vi "DataAcquisitionCode.vi"() -> ()   [LabVIEW 2020]
uses:
  globalvariables.vi
  <vilib>/Utility/file.llb/Read Delimited Spreadsheet (DBL).vi
panel:
  in  "ThM 4":enum32{"Page 1"}(tab)
  out "T-By In 4":dbl
  out "T-Hx In 4":dbl
  out "T-Supply 4":dbl
  out "P-Return 4":dbl
  out "T-Hx Out 4":dbl
  out "P-Hx Out 4":dbl
  out "T-By Out 4":dbl
  out "T-Return 4":dbl
  out "T-PJ Hot 4":dbl
  out "T-PJ Cold 4":dbl
  out "T-ThM 4":dbl(graph)
  out "P-Hx In 4":dbl
  out "P-By In 4":dbl
  out "M-Supply 4":dbl
  in  "ThM 3":enum32{"Page 1"}(tab)
  out "P-By In 3":dbl
  out "P-Hx In 3":dbl
  out "T-ThM 3":dbl(graph)
  out "T-PJ Cold 3":dbl
  out "T-PJ Hot 3":dbl
  out "T-Return 3":dbl
  out "T-By Out 3":dbl
  out "P-Return 3":dbl
  out "T-Hx Out 3":dbl
  out "P-Hx Out 3":dbl
  out "T-Supply 3":dbl
  out "T-By In 3":dbl
  out "T-Hx In 3":dbl
  out "M-Supply 3":dbl
  in  "ThM 1":enum32{"Page 1"}(tab)
  out "M-By 1":dbl format="%.2g"
  out "T-PJ Hot 1":dbl format="%.1g"
  out "T-PJ Cold 1":dbl format="%.1g"
  out "P-Hx Out 1":dbl format="%.2g"
  out "P-Hx In 1":dbl format="%.2g"
  out "P-By In 1":dbl format="%.2g"
  out "T-Hx Out 1":dbl format="%.1g"
  out "T-By Out 1":dbl format="%.1g"
  out "T-By In 1":dbl format="%.1g"
  out "T-Hx In 1":dbl format="%.1g"
  out "T-ThM 1":dbl(graph)
  in  "ThM 2":enum32{"Page 1"}(tab)
  out "M-By 2":dbl format="%.2g"
  out "T-Hx In 2":dbl format="%.1g"
  out "T-By In 2":dbl format="%.1g"
  out "T-Supply 2":dbl format="%.1g"
  out "P-Return 2":dbl format="%.2g"
  out "T-Return 2":dbl format="%.1g"
  out "P-Hx Out 2":dbl format="%.2g"
  out "T-By Out 2":dbl format="%.1g"
  out "T-Hx Out 2":dbl format="%.1g"
  out "T-PJ Hot 2":dbl format="%.1g"
  out "T-PJ Cold 2":dbl format="%.1g"
  out "T-ThM 2":dbl(graph)
  out "P-Hx In 2":dbl format="%.2g"
  out "P-By In 2":dbl format="%.2g"
  out "M-Supply 2":dbl format="%.2g"
  in  "Source":enum32{"Page 1"}(tab)
  out "T-Ambient":dbl format="%.1g"
  out "P-Pump In":dbl format="%.2g"
  out "T-Pump In":dbl format="%.1g"
  out "P-Heater Out":dbl format="%.2g"
  out "T-Heater Out":dbl format="%.1g"
  out "P-Heater In":dbl format="%.2g"
  out "M-Heater":dbl format="%.2g"
  out "T-Heater":dbl format="%.1g"
  in  "Heater Warning":enum32{"Page 1", "Page 2"}(tab)
  in  "Peltier Control Menu":enum32{"Cold Side", "Power"}(tab) caption="Peltier Control"
  in  "Run Peltier M":bool caption="Run"
  in  "Peltier Set Temp In":dbl[](array[slide]) step=0.1 scale=0.0..25.0
  in  "Peltier Update Rate":dbl=60.0 caption="Update Rate (s)"
  in  "Peltier Tamb In":dbl
  in  "Peltier Set Power":dbl[](array[numeric]) caption="Power Setpoint" format="%#.1f"
  out "Peltier Set Temp":dbl[](array[numeric]) caption="Control Temp" format="%#.1g"
  in  "Valve Control Menu":enum32{"Position", "PID"}(tab)
  in  "Run Valve M":bool caption="Run"
  in  "Valve Position Set":dbl[](array[knob]) min=0.0 max=100.0 step=0.1 scale=0.0..100.0
  in  "Valve Update Rate":dbl=60.0 caption="Update Rate (s)"
  in  "Valve Temp Setpoint":dbl[](array[numeric]) caption="Temp Setpoint"
  out "Valve Position":dbl[](array[numeric]) caption="Position"
  in  "Gain":cluster{"P":dbl, "I":dbl, "D":dbl}[](array[cluster]) caption="Gains"
  out "Time Elapsed (s)":dbl format="%#.0f"
  out "Time Limit (s)":dbl
  out "Current Save Directory":path
  out "# of Quick Restarts":i32
  out "# of Data Points Queued":i32
  out "Processing\nData":bool
  out "Acquiring\nData":bool
  in  "Stop Data Acquisition":bool
  # "Thermal Mass 4"
  # "Thermal Mass 3"
  # "Thermal Mass 1"
  # "Thermal Mass 2"
  # "Pump"
  # "Water Heater"
  # "WARNING:\nThe boiler has exceeded 90°C. Abort testing immediately."
  # "Peltier 1"
  # "Peltier 2"
  # "Valve 1"
  # "Valve 2"
  # "Valve 1"
  # "Valve 2"
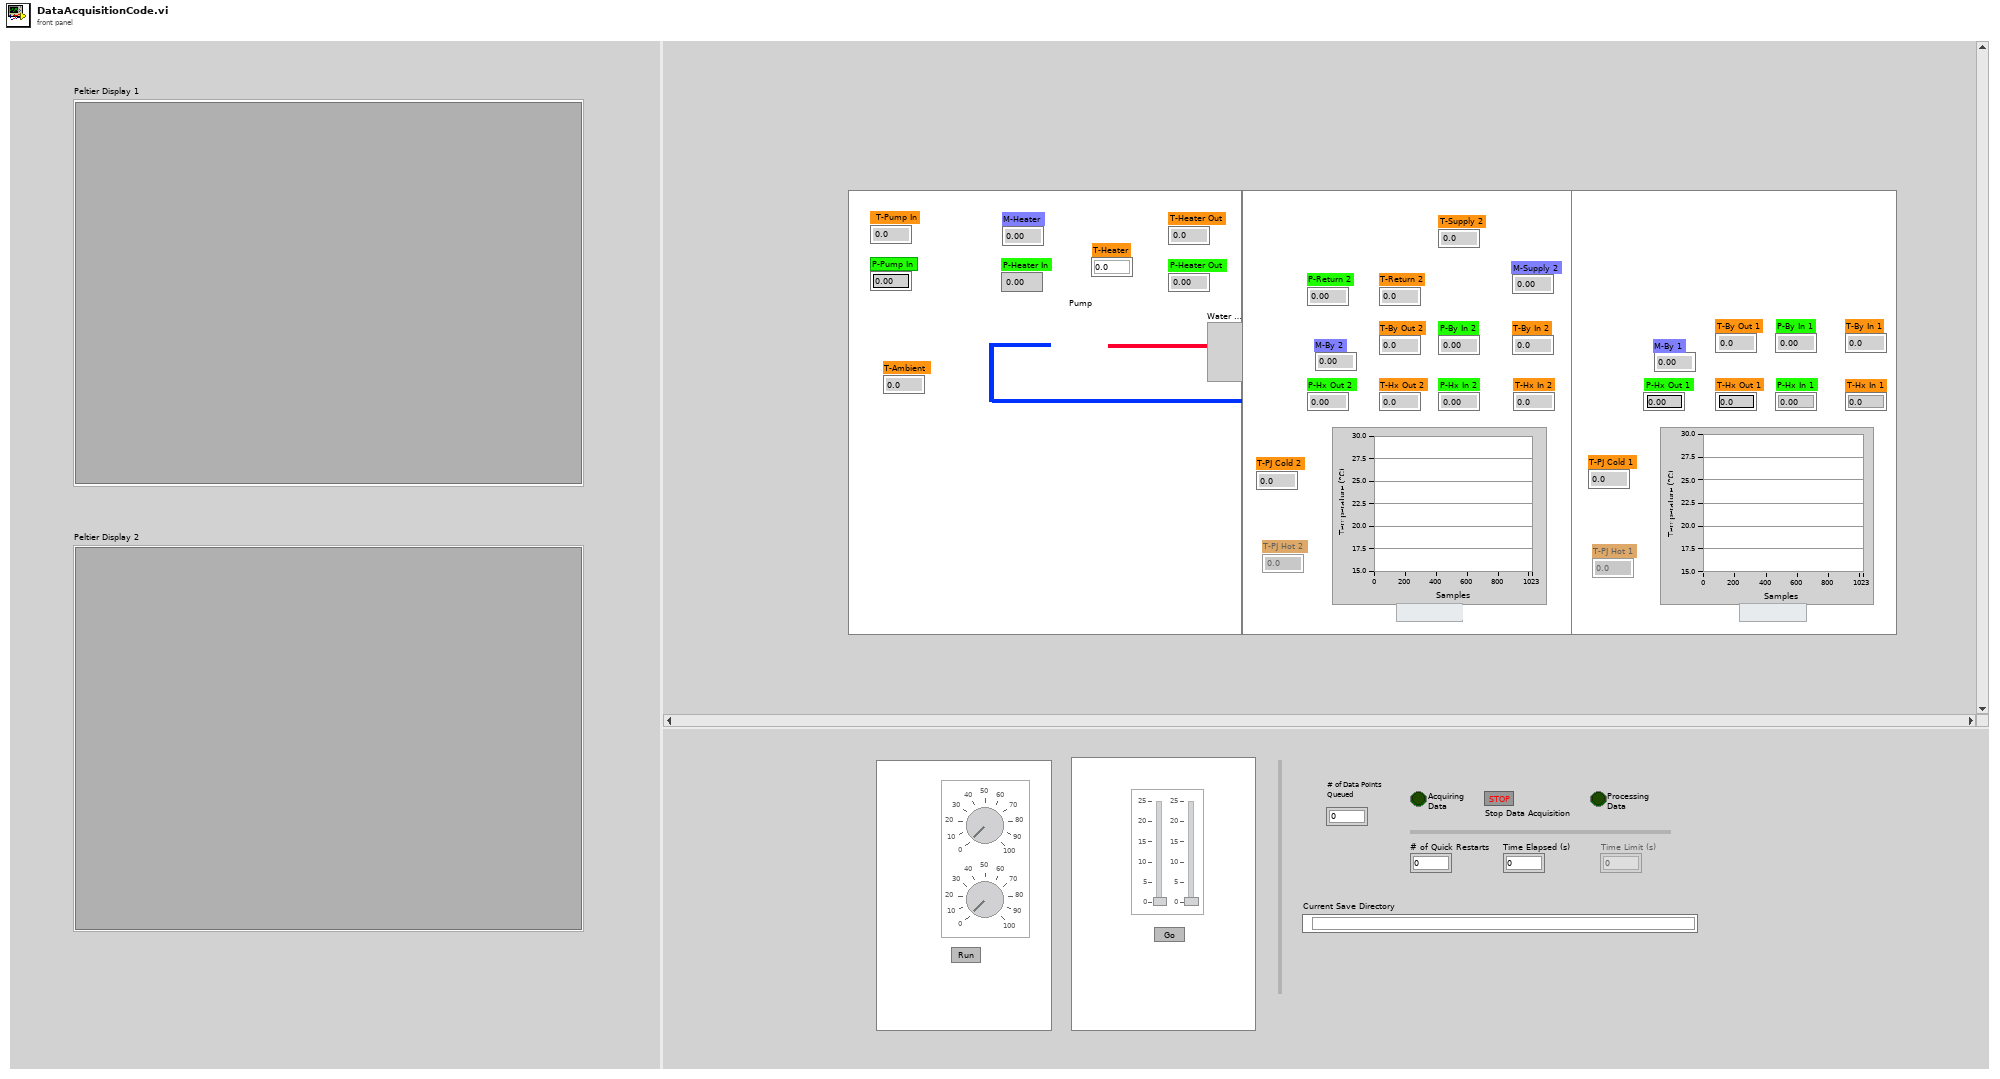
[diagram p1: front panel]
types:
  T1 = cluster{"Omega task":refnum<k24>[], "Sensor task":refnum<k21>, "Actuator task":refnum<k21>, "Omega error":errorcluster[], "Sensor error":errorcluster, "Actuator error":errorcluster}
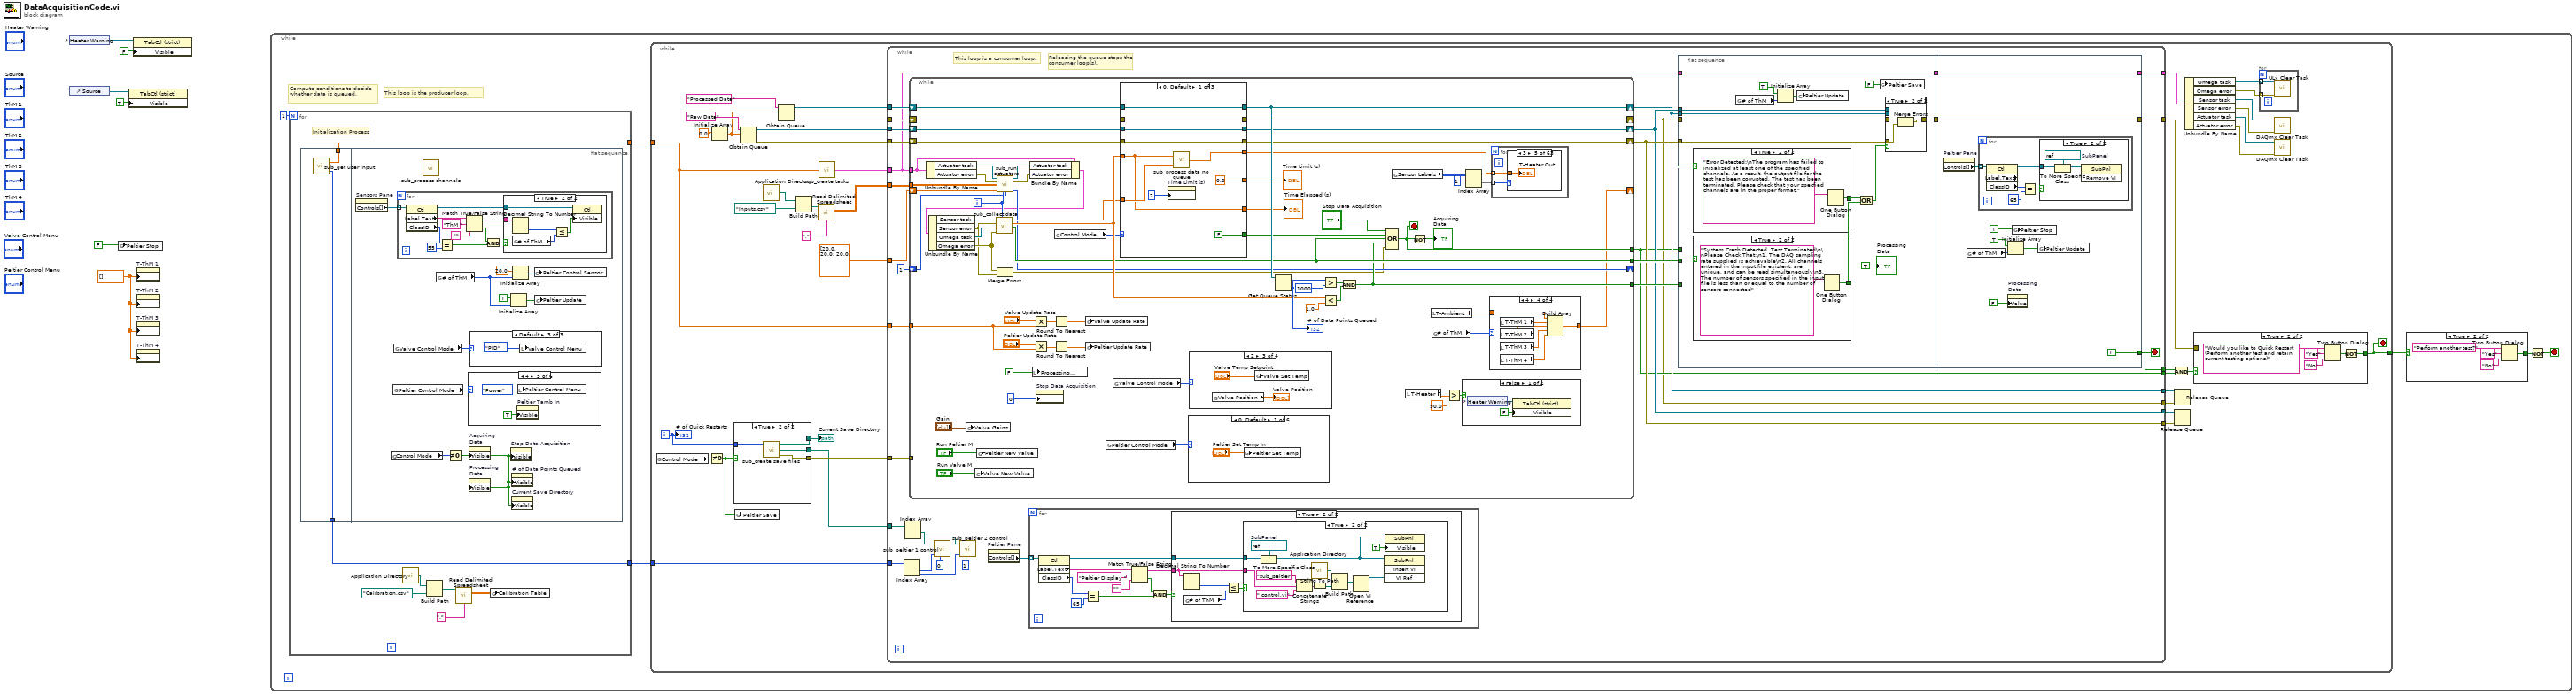
[diagram p0: block diagram]
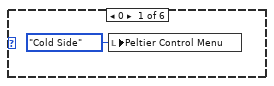
[diagram p3: hidden frame]
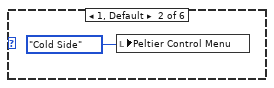
[diagram p4: hidden frame]
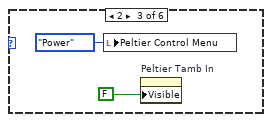
[diagram p5: hidden frame]
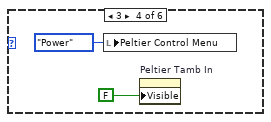
[diagram p6: hidden frame]
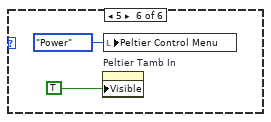
[diagram p7: hidden frame]
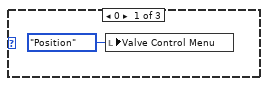
[diagram p8: hidden frame]
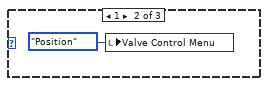
[diagram p9: hidden frame]
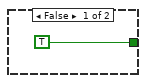
[diagram p10: hidden frame]
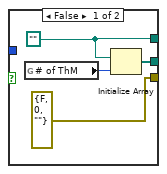
[diagram p11: hidden frame]
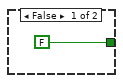
[diagram p12: hidden frame]
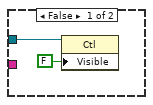
[diagram p14: hidden frame]
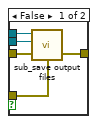
[diagram p15: hidden frame]
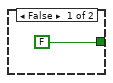
[diagram p16: hidden frame]
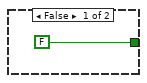
[diagram p17: hidden frame]
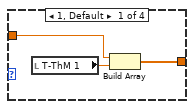
[diagram p19: hidden frame]
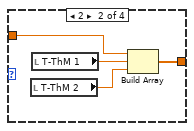
[diagram p20: hidden frame]
diagram:
  w2 = dbl[] []
  n1 = control-ref of="Heater Warning"() -> (w5:refnum<vi>)
  n2 = control-ref of="Source"() -> (w4:refnum<vi>)
  n3 = global write "globalvariables.vi" "Peltier Stop"(FALSE) -> ()
  n4 = property on="Property Node" class="TabCtl (strict)"(reference=w4, "Visible"=TRUE) -> ()  [unwired: 1 in, 2 out]
  n5 = property on="Property Node" class="TabCtl (strict)"(reference=w5, "Visible"=FALSE) -> ()  [unwired: 1 in, 2 out]
  n6 = property on="T-ThM 1" class="WFChart (strict)"("History Data"=w2) -> ()  [unwired: 2 in, 2 out]
  n7 = property on="T-ThM 2" class="WFChart (strict)"("History Data"=w2) -> ()  [unwired: 2 in, 2 out]
  n8 = property on="T-ThM 3" class="WFChart (strict)"("History Data"=w2) -> ()  [unwired: 2 in, 2 out]
  n9 = property on="T-ThM 4" class="WFChart (strict)"("History Data"=w2) -> ()  [unwired: 2 in, 2 out]
  n10 = while {
    stop <- w11 stop-if-true
    # "Compute conditions to decide whether data is queued."
    # "This loop is the producer loop."
    n11 = for {
      N: 1 -> [_]
      tunnel: [w19] -> w9
      tunnel: [w13] -> w7
      # "Initialization Process"
      n12 = flat-sequence {
        tunnel: [w21] -> w19
        tunnel: [w20] -> w13
        frame #0 {
          n13 = call "sub_get user input.vi"() -> ("Peltier Channels"=w20:i16[], "DAQ Sample Rate"=w21:dbl)  [unwired: 2 in]
        }
        frame #1 {
          n14 = property on="Sensors Pane" class="Pane"() -> ("Controls[]"=w22:refnum<vi>[])  [unwired: 2 in, 2 out]
          n15 = global read "globalvariables.vi" "Control Mode"() -> (w28:i32)
          n16 = global read "globalvariables.vi" "Peltier Control Mode"() -> (w30:i16)
          n17 = global read "globalvariables.vi" "Valve Control Mode"() -> (w31:i16)
          n18 = for {
            tunnel: w22 -> [w40] mode=indexing
            n19 = property class="Ctl"(reference=w40) -> (reference out=w41:refnum<vi>, "Label.Text"=w39:string, "ClassID"=w42:u32)  [unwired: 1 in, 1 out]
            n20 = Equal?(x=w42, y=u32 55) -> (x = y?=w32:bool)
            n21 = Match True/False String(2:"", 3:"ThM " ("true string"), 4:w39) -> (0:w33:bool, 1:w35:string)
            n22 = And(x=w33, y=w32) -> (x .and. y?=w34:bool)
            n23 = case shown="True" w34 {
              tunnel: w41 -> [_ w47]
              tunnel: w35 -> [_ w46]
              frame False {
              }
              frame True {
                n24 = global read "globalvariables.vi" "# of ThM"() -> (w43:i32)
                n25 = Decimal String To Number(string=w46) -> (number=w44:i32)  [unwired: 2 in, 1 out]
                n26 = Less Or Equal?(x=w44, y=w43) -> (x <= y?=w45:bool)
                n27 = property class="Ctl"(reference=w47, "Visible"=w45) -> ()  [unwired: 1 in, 2 out]
              }
            }
          }
          n28 = call "sub_process channels.vi"() -> ()  [unwired: 6 in]
          n29 = global read "globalvariables.vi" "# of ThM"() -> (w24:i32)
          n30 = Not Equal To 0?(x=w28) -> (x != 0?=w29:bool)
          n31 = case shown="4" w30 {
            frame 0 {
              n32 = local write "Peltier Control Menu"(enum32{"Cold Side", "Power"}."Cold Side" ("Peltier Control Menu")) -> ()
            }
            frame 1, Default {
              n33 = local write "Peltier Control Menu"(enum32{"Cold Side", "Power"}."Cold Side" ("Peltier Control Menu")) -> ()
            }
            frame 2 {
              n34 = local write "Peltier Control Menu"(enum32{"Cold Side", "Power"}."Power" ("Peltier Control Menu")) -> ()
              n35 = property on="Peltier Tamb In" class="DigNum (strict)"("Visible"=FALSE) -> ()  [unwired: 2 in, 2 out]
            }
            frame 3 {
              n36 = local write "Peltier Control Menu"(enum32{"Cold Side", "Power"}."Power" ("Peltier Control Menu")) -> ()
              n37 = property on="Peltier Tamb In" class="DigNum (strict)"("Visible"=FALSE) -> ()  [unwired: 2 in, 2 out]
            }
            frame 4 {
              n38 = property on="Peltier Tamb In" class="DigNum (strict)"("Visible"=TRUE) -> ()  [unwired: 2 in, 2 out]
              n39 = local write "Peltier Control Menu"(enum32{"Cold Side", "Power"}."Power" ("Peltier Control Menu")) -> ()
            }
            frame 5 {
              n40 = property on="Peltier Tamb In" class="DigNum (strict)"("Visible"=TRUE) -> ()  [unwired: 2 in, 2 out]
              n41 = local write "Peltier Control Menu"(enum32{"Cold Side", "Power"}."Power" ("Peltier Control Menu")) -> ()
            }
          }
          n42 = property on="Acquiring\nData" class="Bool (strict)"("Visible"=w29) -> ()  [unwired: 2 in, 2 out]
          n43 = property on="Processing\nData" class="Bool (strict)"("Visible"=w29) -> ()  [unwired: 2 in, 2 out]
          n44 = case shown="Default" w31 {
            frame 0 {
              n45 = local write "Valve Control Menu"(enum32{"Position", "PID"}."Position" ("Valve Control Menu")) -> ()
            }
            frame 1 {
              n46 = local write "Valve Control Menu"(enum32{"Position", "PID"}."Position" ("Valve Control Menu")) -> ()
            }
            frame Default {
              n47 = local write "Valve Control Menu"(enum32{"Position", "PID"}."PID" ("Valve Control Menu")) -> ()
            }
          }
          n48 = Initialize Array(TRUE, w24) -> (w23:bool[])
          n49 = property on="Stop Data Acquisition" class="Bool"("Visible"=w29) -> ()  [unwired: 2 in, 2 out]
          n50 = property on="# of Data Points Queued" class="DigNum (strict)"("Visible"=w29) -> ()  [unwired: 2 in, 2 out]
          n51 = property on="Current Save Directory" class="Path"("Visible"=w29) -> ()  [unwired: 2 in, 2 out]
          n52 = Initialize Array(20.0 ("element"), w24) -> (w26:dbl[])
          n53 = global write "globalvariables.vi" "Peltier Control Sensor"(w26) -> ()
          n54 = global write "globalvariables.vi" "Peltier Update"(w23) -> ()
        }
      }
      n55 = call <vilib>:"Application Directory.vi"() -> ("Application Directory"=w17:path)
      n56 = Build Path(base path=w17, name or relative path=path "Calibration.csv") -> (appended path=w18:path)
      n57 = call-poly <vilib>:"Read Delimited Spreadsheet.vi"("file path (dialog if empty)"=w18, "delimiter (\\t)"=",") -> ("all rows"=w16:dbl[][])  [unwired: 8 in, 5 out]
      n58 = global write "globalvariables.vi" "Calibration Table"(w16) -> ()
    }
    n59 = while {
      tunnel: [w99] -> w10
      tunnel: w9 -> [w92]
      tunnel: w7 -> [w67]
      i -> [w90]
      stop <- w99 stop-if-true
      n60 = global read "globalvariables.vi" "Control Mode"() -> (w88:i32)
      n61 = Not Equal To 0?(x=w88) -> (x != 0?=w87:bool)
      n62 = Initialize Array(0.0) -> (w84:dbl[])  [unwired: 1 in]
      n63 = case shown="True" w87 {
        tunnel: w90 -> [_ w112]
        tunnel: [w108 w111] -> w73
        tunnel: [errorcluster {"status"=FALSE, "code"=0, "source"=""} ("error constant") w110] -> w86
        tunnel: [w105 w109] -> w81
        frame False {
          w105 = path ""
          n64 = global read "globalvariables.vi" "# of ThM"() -> (w107:i32)
          n65 = Initialize Array(w105, w107) -> (w108:path[])
        }
        frame True {
          n66 = call "sub_create save files.vi"("# of Quick Restarts"=w112) -> ("error out"=w110:errorcluster, "Peltier Save Files"=w111:path[], "Save Path"=w109:path)  [unwired: 2 in]
        }
      }
      "Current Save Directory" <- w81
      n67 = global write "globalvariables.vi" "Peltier Save"(w87) -> ()
      n68 = Obtain Queue(name (unnamed)="Raw Data", element data type=w84) -> (queue out=w96:refnum<queue>, error out=w95:errorcluster)  [unwired: 3 in, 1 out]
      n69 = call <vilib>:"Application Directory.vi"() -> ("Application Directory"=w69:path)
      n70 = Obtain Queue(name (unnamed)="Processed Data", element data type=w84) -> (queue out=w102:refnum<queue>, error out=w101:errorcluster)  [unwired: 3 in, 1 out]
      n71 = Build Path(base path=w69, name or relative path=path "Inputs.csv") -> (appended path=w70:path)
      n72 = call-poly <vilib>:"Read Delimited Spreadsheet.vi"("file path (dialog if empty)"=w70, "delimiter (\\t)"=",") -> ("all rows"=w68:dbl[][])  [unwired: 8 in, 5 out]
      n73 = call "sub_create tasks.vi"("DAQ Sample Rate"=w92) -> ("output cluster"=w89:T1)
      n74 = while {
        tunnel: [w140] -> w104
        tunnel: [w132] -> w103
        tunnel: w102 -> [w150]
        tunnel: w101 -> [w151]
        tunnel: [w139] -> w91
        tunnel: w96 -> [w148]
        tunnel: w95 -> [w149]
        tunnel: [w141] -> w94
        tunnel: [w143] -> w93
        tunnel: w92 -> [w146]
        tunnel: w89 -> [w134]
        tunnel: [w133] -> w80
        tunnel: w86 -> [w142]
        tunnel: [w138] -> w83
        tunnel: [w137] -> w82
        tunnel: w73 -> [w129]
        tunnel: w68 -> [w131]
        tunnel: w67 -> [w128]
        tunnel: dbl[] [20.0, 20.0, 20.0] -> [w121]
        stop <- w138 stop-if-true
        # "This loop is a consumer loop."
        # "Releasing the queue stops the consumer loop(s)."
        n75 = Index Array(array=w128) -> (element #1=w125:i16, element #2=w124:i16)  [unwired: 2 in]
        n76 = Index Array(array=w129) -> (element #1=w123:path, element #2=w122:path)  [unwired: 2 in]
        n77 = while {
          shift-right: [w277] -> w132
          shift-left: w151 -> [w285]
          shift-right: [w279] -> w140
          shift-left: w150 -> [w283]
          tunnel: [w268] -> w139
          tunnel: [w267] -> w147
          tunnel: w146 -> [w244]
          tunnel: [w269] -> w145
          shift-right: [w259] -> _
          shift-left: 1 -> [w260]
          shift-right: [w273] -> w141
          shift-left: w148 -> [w281]
          shift-right: [w272] -> w143
          shift-left: w149 -> [w280]
          tunnel: w134 -> [w240]
          shift-right: [w246] -> _
          shift-left: w121 -> [w258]
          tunnel: w142 -> [_]
          tunnel: w131 -> [w234]
          i -> [w261]
          stop <- w268 stop-if-true
          n78 = Unbundle By Name(w240) -> ("Actuator task"=w242:refnum<k21>, "Actuator error"=w241:errorcluster)
          n79 = global write "globalvariables.vi" "Valve Gains"("Gain") -> ()
          n80 = global write "globalvariables.vi" "Valve New Value"("Run Valve M") -> ()
          n81 = global write "globalvariables.vi" "Peltier New Value"("Run Peltier M") -> ()
          n82 = call "sub_run actuators.vi"("Actuator Task"=w242, "Actuator error"=w241, "Inputs"=w234, "T_control"=w258, "Iteration"=w261, "Control Counter in"=w260) -> ("task out"=w239:refnum<k21>, "error out"=w238:errorcluster, "Control Counter out"=w259:i32)  [unwired: 7 in]
          n83 = Bundle By Name(cluster=w240, "Actuator task"=w239, "Actuator error"=w238) -> (w237:T1)
          n84 = Unbundle By Name(w237) -> ("Sensor task"=w236:refnum<k21>, "Sensor error"=w231:errorcluster, "Omega task"=w235:refnum<k24>[], "Omega error"=w232:errorcluster[])
          n85 = call "sub_collect data.vi"("Iteration"=w261, "Omega error"=w232, "Omega task"=w235, "Sensor error"=w231, "Sensor Task"=w236) -> ("All initialized?"=w269:bool, "Elapsed Time (s)"=w284:dbl, "Sensor Data"=w282:dbl[])  [unwired: 4 in]
          n86 = Merge Errors(w232, w231) -> (w230:errorcluster)
          n87 = local write "Processing\nData"(FALSE) -> ()
          n88 = Multiply(x="Valve Update Rate", y=w244) -> (x*y=w255:dbl)
          n89 = Multiply(x="Peltier Update Rate", y=w244) -> (x*y=w252:dbl)
          n90 = property on="Stop Data Acquisition" class="Bool"("DisabledEnum"=0) -> ()  [unwired: 2 in, 2 out]
          n91 = Round To Nearest(number=w255) -> (nearest integer value=w254:dbl)
          n92 = Round To Nearest(number=w252) -> (nearest integer value=w250:dbl)
          n93 = global read "globalvariables.vi" "Control Mode"() -> (w257:i32)
          n94 = global write "globalvariables.vi" "Valve Update Rate"(w254) -> ()
          n95 = global write "globalvariables.vi" "Peltier Update Rate"(w250) -> ()
          n96 = global read "globalvariables.vi" "Peltier Control Mode"() -> (w248:i16)
          n97 = global read "globalvariables.vi" "Valve Control Mode"() -> (w249:i16)
          n98 = case shown="0, Default" w257 {
            tunnel: [w406 w420 w432] -> w279
            tunnel: w285 -> [w405 w419 w431]
            tunnel: [w405 w418 w433] -> w277
            tunnel: w284 -> [w397 w407 w421]
            tunnel: w283 -> [w406 w417 w434]
            tunnel: [FALSE FALSE w423] -> w264
            tunnel: w282 -> [w399 w416 w430]
            tunnel: w281 -> [w404 w415 w429]
            tunnel: w280 -> [w403 w414 w428]
            tunnel: [w404 w413 w427] -> w273
            tunnel: [w403 w412 w426] -> w272
            tunnel: [w398 w411 w425] -> w243
            tunnel: [0.0 0.0 w422] -> w266
            tunnel: [w397 w407 w421] -> w265
            frame 0, Default {
              n99 = property on="Time Limit (s)" class="DigNum (strict)"("DisabledEnum"=2) -> ()  [unwired: 2 in, 2 out]
              n100 = call "sub_process data no queue.vi"("Raw Data"=w399, "Elapsed Time (s)"=w397) -> ("Processed Data"=w398:dbl[])
            }
            frame 1 {
              n101 = call "sub_process data.vi"("Processed Queue in"=w417, "Elapsed Time (s)"=w407, "Processed error in"=w419, "Raw Queue in"=w415, "Raw error in"=w414, "Raw Data in"=w416) -> ("Processed Queue out"=w420:refnum<queue>, "Processed error out"=w418:errorcluster, "Raw Queue out"=w413:refnum<queue>, "Processed Data Out"=w411:dbl[], "Raw error out"=w412:errorcluster)  [unwired: 5 in]
              n102 = property on="Time Limit (s)" class="DigNum (strict)"("DisabledEnum"=2) -> ()  [unwired: 2 in, 2 out]
            }
            frame 2 {
              n103 = global read "globalvariables.vi" "Timer Length"() -> (w422:dbl)
              n104 = property on="Time Limit (s)" class="DigNum (strict)"("DisabledEnum"=0) -> ()  [unwired: 2 in, 2 out]
              n105 = call "sub_process data.vi"("Processed Queue in"=w434, "Elapsed Time (s)"=w421, "Processed error in"=w431, "Raw Queue in"=w429, "Raw error in"=w428, "Raw Data in"=w430) -> ("Processed Queue out"=w432:refnum<queue>, "Processed error out"=w433:errorcluster, "Raw Queue out"=w427:refnum<queue>, "Processed Data Out"=w425:dbl[], "Raw error out"=w426:errorcluster)  [unwired: 5 in]
              n106 = Greater Or Equal?(x=w421, y=w422) -> (x >= y?=w423:bool)
            }
          }
          "Time Limit (s)" <- w266
          "Time Elapsed (s)" <- w265
          n107 = case shown="0, Default" w248 {
            frame 0, Default {
              n108 = global write "globalvariables.vi" "Peltier Set Temp"("Peltier Set Temp In") -> ()
            }
            frame 1 {
              n109 = global read "globalvariables.vi" "Peltier Set Temp"() -> (w312:dbl[])
              n110 = local write "Peltier Set Temp In"(w312) -> ()
            }
            frame 2 {
              n111 = global read "globalvariables.vi" "Peltier Set Temp"() -> (→"Peltier Set Temp":dbl[])
              n112 = global write "globalvariables.vi" "Peltier Set Power"("Peltier Set Power") -> ()
            }
            frame 3 {
              n113 = global read "globalvariables.vi" "Peltier Set Power"() -> (w315:dbl[])
              n114 = global read "globalvariables.vi" "Peltier Set Temp"() -> (w316:dbl[])
              n115 = local write "Peltier Set Temp"(w316) -> ()
              n116 = local write "Peltier Set Power"(w315) -> ()
            }
            frame 4 {
              n117 = global read "globalvariables.vi" "Peltier Set Power"() -> (w318:dbl[])
              n118 = global read "globalvariables.vi" "Peltier Set Temp"() -> (w317:dbl[])
              n119 = local write "Peltier Set Power"(w318) -> ()
              n120 = local write "Peltier Set Temp"(w317) -> ()
              n121 = global write "globalvariables.vi" "Peltier Tamb"("Peltier Tamb In") -> ()
            }
            frame 5 {
              n122 = global read "globalvariables.vi" "Peltier Set Power"() -> (w320:dbl[])
              n123 = global read "globalvariables.vi" "Peltier Set Temp"() -> (w321:dbl[])
              n124 = global read "globalvariables.vi" "Peltier Tamb"() -> (w322:dbl)
              n125 = local write "Peltier Set Power"(w320) -> ()
              n126 = local write "Peltier Set Temp"(w321) -> ()
              n127 = local write "Peltier Tamb In"(w322) -> ()
            }
          }
          n128 = case shown="2" w249 {
            frame 0, Default {
              n129 = global write "globalvariables.vi" "Valve Position"("Valve Position Set") -> ()
            }
            frame 1 {
              n130 = global read "globalvariables.vi" "Valve Position"() -> (w324:dbl[])
              n131 = local write "Valve Position Set"(w324) -> ()
            }
            frame 2 {
              n132 = global read "globalvariables.vi" "Valve Position"() -> (→"Valve Position":dbl[])
              n133 = global write "globalvariables.vi" "Valve Set Temp"("Valve Temp Setpoint") -> ()
            }
            frame 3 {
              n134 = global read "globalvariables.vi" "Valve Set Temp"() -> (w327:dbl[])
              n135 = global read "globalvariables.vi" "Valve Position"() -> (w328:dbl[])
              n136 = local write "Valve Temp Setpoint"(w327) -> ()
              n137 = local write "Valve Position"(w328) -> ()
            }
          }
          n138 = Get Queue Status(queue=w279) -> (# elements in queue=w288:i32)  [unwired: 2 in, 7 out]
          "# of Data Points Queued" <- w288
          n139 = Greater?(x=w288, y=1000) -> (0:w290:bool)
          n140 = Less?(x=w284, y=1.0) -> (x < y?=w286:bool)
          n141 = And(x=w290, y=w286) -> (x .and. y?=w267:bool)
          n142 = Compound Arithmetic op=OR("Stop Data Acquisition", w264, w269, w267, w230) -> (w268:bool)
          n143 = global read "globalvariables.vi" "Sensor Labels"() -> (w270:i32[][])
          n144 = local read "T-Heater"() -> (w275:dbl)
          n145 = Not(x=w268) -> (.not. x?=→"Acquiring\nData":bool)
          n146 = local read "T-Ambient"() -> (w233:dbl)
          n147 = global read "globalvariables.vi" "# of ThM"() -> (w247:i32)
          n148 = Greater?(x=w275, y=90.0) -> (0:w278:bool)
          n149 = case shown="False" w278 {
            frame False {
              n150 = control-ref of="Heater Warning"() -> (w393:refnum<vi>)
              n151 = property on="Property Node" class="TabCtl (strict)"(reference=w393, "Visible"=FALSE) -> ()  [unwired: 1 in, 2 out]
            }
            frame True {
              n152 = control-ref of="Heater Warning"() -> (w395:refnum<vi>)
              n153 = property on="Property Node" class="TabCtl (strict)"(reference=w395, "Visible"=TRUE) -> ()  [unwired: 1 in, 2 out]
            }
          }
          n154 = Index Array(array=w270, index (row)=1) -> (element=w245:i32[])  [unwired: 1 in]
          n155 = case shown="4" w247 {
            tunnel: [w295 w299 w304 w310] -> w246
            tunnel: w233 -> [w293 w296 w300 w305]
            frame 1, Default {
              n156 = local read "T-ThM 1"() -> (w294:dbl)
              n157 = Build Array(w293, w294) -> (w295:dbl[])
            }
            frame 2 {
              n158 = local read "T-ThM 2"() -> (w297:dbl)
              n159 = local read "T-ThM 1"() -> (w298:dbl)
              n160 = Build Array(w296, w298, w297) -> (w299:dbl[])
            }
            frame 3 {
              n161 = local read "T-ThM 3"() -> (w301:dbl)
              n162 = local read "T-ThM 1"() -> (w303:dbl)
              n163 = local read "T-ThM 2"() -> (w302:dbl)
              n164 = Build Array(w300, w303, w302, w301) -> (w304:dbl[])
            }
            frame 4 {
              n165 = local read "T-ThM 1"() -> (w306:dbl)
              n166 = local read "T-ThM 2"() -> (w307:dbl)
              n167 = local read "T-ThM 3"() -> (w308:dbl)
              n168 = local read "T-ThM 4"() -> (w309:dbl)
              n169 = Build Array(w305, w306, w307, w308, w309) -> (w310:dbl[])
            }
          }
          n170 = for {
            tunnel: w243 -> [w329] mode=indexing
            tunnel: w245 -> [w330] mode=indexing
            n171 = case shown="3" w330 {
              tunnel: w329 -> [_ w331 w332 w333 w334 w335 w336 w337 w338 w339 w340 w341 w342 w343 w344 w345 w346 w347 w348 w349 w350 w351 w352 w353 w354 w355 w356 w357 w358 w359 w360 w361 w362 w363 w364 w365 w366 w367 w368 w369 w370 w371 w372 w373 w374 w375 w376 w377 w378 w379 w380 w381 w382 w383 w384 w385 w386 w387 w388 w389 w390 w391 w392]
              frame Default {
              }
              frame 0 {
                "T-Ambient" <- w331
              }
              frame 1 {
                "T-Pump In" <- w332
              }
              frame 2 {
                "T-Heater" <- w333
              }
              frame 3 {
                "T-Heater Out" <- w334
              }
              frame 4 {
                "P-Pump In" <- w335
              }
              frame 5 {
                "P-Heater In" <- w336
              }
              frame 6 {
                "P-Heater Out" <- w337
              }
              frame 7 {
                "M-Heater" <- w338
              }
              frame 8 {
                "T-By In 1" <- w339
              }
              frame 9 {
                "T-Hx In 1" <- w340
              }
              frame 10 {
                "T-PJ Cold 1" <- w341
              }
              frame 11 {
                "T-PJ Hot 1" <- w342
              }
              frame 12 {
                "T-Hx Out 1" <- w343
              }
              frame 13 {
                "T-By Out 1" <- w344
              }
              frame 14 {
                "P-By In 1" <- w345
              }
              frame 15 {
                "P-Hx In 1" <- w346
              }
              frame 16 {
                "P-Hx Out 1" <- w347
              }
              frame 17 {
                "T-ThM 1" <- w348
              }
              frame 18 {
                "T-Supply 2" <- w349
              }
              frame 19 {
                "T-By In 2" <- w350
              }
              frame 20 {
                "T-Hx In 2" <- w351
              }
              frame 21 {
                "T-PJ Cold 2" <- w352
              }
              frame 22 {
                "T-PJ Hot 2" <- w353
              }
              frame 23 {
                "T-Hx Out 2" <- w354
              }
              frame 24 {
                "T-By Out 2" <- w355
              }
              frame 25 {
                "T-Return 2" <- w356
              }
              frame 26 {
                "P-By In 2" <- w357
              }
              frame 27 {
                "P-Hx In 2" <- w358
              }
              frame 28 {
                "P-Hx Out 2" <- w359
              }
              frame 29 {
                "P-Return 2" <- w360
              }
              frame 30 {
                "M-Supply 2" <- w361
              }
              frame 31 {
                "T-ThM 2" <- w362
              }
              frame 32 {
                "T-Supply 3" <- w363
              }
              frame 33 {
                "T-By In 3" <- w364
              }
              frame 34 {
                "T-Hx In 3" <- w365
              }
              frame 35 {
                "T-PJ Cold 3" <- w366
              }
              frame 36 {
                "T-PJ Hot 3" <- w367
              }
              frame 37 {
                "T-Hx Out 3" <- w368
              }
              frame 38 {
                "T-By Out 3" <- w369
              }
              frame 39 {
                "T-Return 3" <- w370
              }
              frame 40 {
                "P-By In 3" <- w371
              }
              frame 41 {
                "P-Hx In 3" <- w372
              }
              frame 42 {
                "P-Hx Out 3" <- w373
              }
              frame 43 {
                "P-Return 3" <- w374
              }
              frame 44 {
                "M-Supply 3" <- w375
              }
              frame 45 {
                "T-ThM 3" <- w376
              }
              frame 46 {
                "T-Supply 4" <- w377
              }
              frame 47 {
                "T-By In 4" <- w378
              }
              frame 48 {
                "T-Hx In 4" <- w379
              }
              frame 49 {
                "T-PJ Cold 4" <- w380
              }
              frame 50 {
                "T-PJ Hot 4" <- w381
              }
              frame 51 {
                "T-Hx Out 4" <- w382
              }
              frame 52 {
                "T-By Out 4" <- w383
              }
              frame 53 {
                "T-Return 4" <- w384
              }
              frame 54 {
                "P-By In 4" <- w385
              }
              frame 55 {
                "P-Hx In 4" <- w386
              }
              frame 56 {
                "P-Hx Out 4" <- w387
              }
              frame 57 {
                "P-Return 4" <- w388
              }
              frame 58 {
                "M-Supply 4" <- w389
              }
              frame 59 {
                "T-ThM 4" <- w390
              }
              frame 60 {
                "M-By 1" <- w391
              }
              frame 61 {
                "M-By 2" <- w392
              }
            }
          }
        }
        n172 = call "sub_peltier 1 control.vi"("Save File"=w123, "COM"=w125, "Array #"=0) -> ()  [unwired: 3 in]
        n173 = call "sub_peltier 2 control.vi"("Save File"=w122, "COM"=w124, "Array #"=1) -> ()  [unwired: 3 in]
        n174 = property on="Peltier Pane" class="Pane"() -> ("Controls[]"=w130:refnum<vi>[])  [unwired: 2 in, 2 out]
        n175 = for {
          tunnel: w130 -> [w159] mode=indexing
          n176 = property class="Ctl"(reference=w159) -> (reference out=w160:refnum<vi>, "Label.Text"=w158:string, "ClassID"=w162:u32)  [unwired: 1 in, 1 out]
          n177 = Equal?(x=w162, y=u32 65) -> (x = y?=w152:bool)
          n178 = Match True/False String(2:"", 3:"Peltier Display " ("true string"), 4:w158) -> (0:w154:bool, 1:w155:string)
          n179 = And(x=w154, y=w152) -> (x .and. y?=w153:bool)
          n180 = case shown="True" w153 {
            tunnel: w160 -> [_ w166]
            tunnel: w155 -> [_ w165]
            frame False {
            }
            frame True {
              n181 = global read "globalvariables.vi" "# of ThM"() -> (w163:i32)
              n182 = Decimal String To Number(string=w165) -> (number=w164:i32)  [unwired: 2 in, 1 out]
              n183 = Less Or Equal?(x=w164, y=w163) -> (x <= y?=w167:bool)
              n184 = case shown="True" w167 {
                tunnel: w166 -> [w169 w171]
                tunnel: w165 -> [_ w177]
                frame False {
                  n185 = property class="Ctl"(reference=w169, "Visible"=FALSE) -> ()  [unwired: 1 in, 2 out]
                }
                frame True {
                  w181 = refnum<vi> refnum  # SubPanel
                  n186 = To More Specific Class(target class=w181, reference=w171) -> (specific class reference=w170:refnum<vi>)  [unwired: 1 in, 1 out]
                  n187 = Concatenate Strings("sub_peltier " ("string"), w177, " control.vi" ("string")) -> (w176:string)
                  n188 = call <vilib>:"Application Directory.vi"() -> ("Application Directory"=w179:path)
                  n189 = String To Path(string=w176) -> (path=w175:path)
                  n190 = Build Path(base path=w179, name or relative path=w175) -> (appended path=w178:path)
                  n191 = Open VI Reference(vi path=w178) -> (vi reference=w172:refnum<vi>)  [unwired: 5 in, 1 out]
                  n192 = invoke class="SubPnl" method="Insert VI"(reference=w170, "VI Ref"=w172) -> ()  [unwired: 2 in, 4 out]
                  n193 = property class="SubPnl"(reference=w170, "Visible"=TRUE) -> ()  [unwired: 1 in, 2 out]
                }
              }
            }
          }
        }
        n194 = flat-sequence {
          tunnel: w132 -> [w197]
          tunnel: w147 -> [w196]
          tunnel: w145 -> [w195]
          tunnel: w143 -> [w194]
          tunnel: w141 -> [w193]
          tunnel: w140 -> [w192]
          tunnel: w139 -> [_]
          tunnel: [w186] -> w136
          tunnel: [w185] -> w135
          tunnel: w134 -> [w185]
          tunnel: [TRUE] -> w138
          tunnel: [w217] -> w137
          tunnel: w136 -> [w217]
          tunnel: [w216] -> w133
          tunnel: w135 -> [w216]
          frame #0 {
            n195 = case shown="True" w196 {
              tunnel: [FALSE w211] -> w190
              frame False {
              }
              frame True {
                n196 = One Button Dialog(message="System Crash Detected. Test Terminated\n\nPlease Check That:\n1. The DAQ sampling rate supplied is achievable\n2. All channels entered in the input file existent, are unique, and can be read simultaneously\n3. The number of sensors specified in the input file is less than or equal to the number of sensors connected") -> (true=w211:bool)  [unwired: 1 in]
              }
            }
            n197 = case shown="True" w195 {
              tunnel: [FALSE w208] -> w191
              frame False {
              }
              frame True {
                n198 = One Button Dialog(message="Error Detected:\nThe program has failed to initialized at least one of the specified channels. As a result, the output file for the test has been corrupted. The test has been terminated. Please check that your specfied channels are in the proper format.") -> (true=w208:bool)  [unwired: 1 in]
              }
            }
            n199 = global read "globalvariables.vi" "# of ThM"() -> (w184:i32)
            n200 = Initialize Array(TRUE, w184) -> (w182:bool[])
            n201 = global write "globalvariables.vi" "Peltier Update"(w182) -> ()
            n202 = Compound Arithmetic op=OR(w191, w190) -> (w188:bool)
            n203 = global write "globalvariables.vi" "Peltier Save"(FALSE) -> ()
            n204 = case shown="True" w188 {
              tunnel: w193 -> [w202 _]
              tunnel: w192 -> [w201 _]
              tunnel: w194 -> [w200 w205]
              tunnel: w197 -> [w199 w204]
              tunnel: [w198 w203] -> w186
              frame False {
                n205 = call "sub_save output files.vi"("Raw Queue in"=w202, "Processed Queue in"=w201, "Raw Data error"=w200, "Processed Data error"=w199) -> ("error out"=w198:errorcluster)  [unwired: 3 in]
              }
              frame True {
                n206 = Merge Errors(w204, w205) -> (w203:errorcluster)
              }
            }
            "Processing\nData" <- TRUE
          }
          frame #1 {
            n207 = property on="Peltier Pane" class="Pane"() -> ("Controls[]"=w215:refnum<vi>[])  [unwired: 2 in, 2 out]
            n208 = global read "globalvariables.vi" "# of ThM"() -> (w214:i32)
            n209 = for {
              tunnel: w215 -> [w222] mode=indexing
              n210 = property class="Ctl" props=["Label", "Text", "ClassID"](reference=w222) -> (reference out=w223:refnum<vi>, "ClassID"=w225:u32)  [unwired: 1 in, 2 out]
              n211 = Equal?(x=w225, y=u32 65) -> (x = y?=w221:bool)
              n212 = case shown="True" w221 {
                tunnel: w223 -> [_ w228]
                frame False {
                }
                frame True {
                  w226 = refnum<vi> refnum  # SubPanel
                  n213 = To More Specific Class(target class=w226, reference=w228) -> (specific class reference=w227:refnum<vi>)  [unwired: 1 in, 1 out]
                  n214 = invoke class="SubPnl" method="Remove VI"(reference=w227) -> ()  [unwired: 2 in, 3 out]
                }
              }
            }
            n215 = Initialize Array(TRUE, w214) -> (w212:bool[])
            n216 = property on="Processing\nData" class="Bool (strict)"("Value"=FALSE) -> ()  [unwired: 2 in, 2 out]
            n217 = global write "globalvariables.vi" "Peltier Stop"(TRUE) -> ()
            n218 = global write "globalvariables.vi" "Peltier Update"(w212) -> ()
          }
        }
      }
      n219 = And(x=w83, y=w91) -> (x .and. y?=w100:bool)
      n220 = Release Queue(queue=w104, error in (no error)=w103) -> ()  [unwired: 1 in, 3 out]
      n221 = Release Queue(queue=w94, error in (no error)=w93) -> ()  [unwired: 1 in, 3 out]
      n222 = Unbundle By Name(w80) -> ("Omega task"=w79:refnum<k24>[], "Omega error"=w78:errorcluster[], "Sensor task"=w77:refnum<k21>, "Sensor error"=w76:errorcluster, "Actuator task"=w75:refnum<k21>, "Actuator error"=w74:errorcluster)
      n223 = case shown="True" w100 {
        tunnel: [FALSE w118] -> w99
        tunnel: w82 -> [_ _]
        frame False {
        }
        frame True {
          n224 = Two Button Dialog(message="Would you like to Quick Restart (Perform another test and retain current testing options)", 1:"No", 2:"Yes") -> (T button?=w119:bool)
          n225 = Not(x=w119) -> (.not. x?=w118:bool)
        }
      }
      n226 = for {
        tunnel: w79 -> [w114] mode=indexing
        tunnel: w78 -> [w113] mode=indexing
        n227 = call <vilib>:"ULx Clear Task.vi"("task in"=w114, "error in"=w113) -> ()  [unwired: 13 in, 1 out]
      }
      n228 = call <vilib>:"DAQmx Clear Task.vi"("task in"=w77, "error in"=w76) -> ()  [unwired: 13 in, 1 out]
      n229 = call <vilib>:"DAQmx Clear Task.vi"("task in"=w75, "error in"=w74) -> ()  [unwired: 13 in, 1 out]
      "# of Quick Restarts" <- w90
    }
    n230 = case shown="True" w10 {
      tunnel: [TRUE w65] -> w12
      frame False {
      }
      frame True {
        n231 = Two Button Dialog(message="Perform another test?", 1:"No", 2:"Yes") -> (T button?=w65:bool)
      }
    }
    n232 = Not(x=w12) -> (.not. x?=w11:bool)
  }
